vi "GUI PS Main Window.vi"() -> ()   [LabVIEW 2011]
uses:
  Types Definitions/Typer GUI PS.ctl
  <vilib>/Platform/TimedLoop/XDataNode/timing_clust.ctl
  <vilib>/Platform/TimedLoop/XDataNode/nitl_modes.ctl
  <vilib>/Platform/TimedLoop/XDataNode/wakeup.ctl
  Types Definitions/Type Configuration Data (GUI to Controller).ctl
  Types Definitions/Type FOFB Parameters.ctl
  Types Definitions/Type Network Configuration.ctl
  Types Definitions/Type FA Configuration.ctl
  Types Definitions/Type Response Matrix Measurement Configuration.ctl
  Types Definitions/Type Correction Algorithm Configuration.ctl
  Types Definitions/Type Acquisition Network Configuration.ctl
  Types Definitions/Type Actuation Network Configuration.ctl
  Types Definitions/Type Configuration Change Acknowledge (Controller to GUI).ctl
  <vilib>/Platform/TimedLoop/XDataNode/XDataNode.xnode
  <vilib>/Platform/TimedLoop/XDataNode/XDNodeRunTimeDep.lvlib
  Type Definitions.lvlib
  LNLS Control VIs.lvlib
  Misc VIs.lvlib
panel:
  in  "Step de corrente (A)":dbl
  in  "Stop Test":bool
  out "Status":bool
  out "error out":errorcluster
  in  "Step Amplitude OK":bool
  in  "Initialize Test":bool
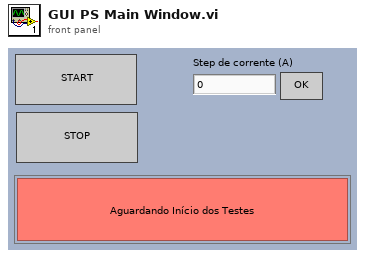
[diagram p1: front panel]
types:
  T1 = enum16{"Idle", "Wait Connection", "Read Data", "Process Data", "Write Data", "Close Connection"}
  T2 = enum16{"Wait Connection", "Read Data", "Write Data", "Close Connection", "Idle"}
  T3 = typedef "Type Definitions.lvlib/Typer GUI PS.ctl" = cluster{"Change Step Value":refnum<notifier>, "Stop VI":refnum<notifier>, "Intialize/Stop Test":refnum<notifier>}
  T4 = typedef "XDNodeRunTimeDep.lvlib/timing_clust.ctl" = cluster{"Expected End [f-1]":u64, "Actual End [f-1]":u64, "Finished Late? [f-1]":bool, "Expected End [i-1]":u64, "Actual End [i-1]":u64, "Finished Late? [i-1]":bool, "Expected Start [i]":u64, "Actual Start [i]":u64, "Expected Start [f]":u64, "Actual Start [f]":u64, "Source Name":string, "Structure Name":string, "Period":i64, "Deadline":i64, "Offset":i64, "Start":i64, "Priority":i32, "Timeout":i32, "Mode":T5, "Wakeup Reason":T6, "Error":errorcluster, "Source Type":string, "Secondary Source Type":string, "Global End Time":u64, "Global Start Time":u64, "Frame Duration":u64, "Iteration Duration":u64, "Assigned CPU":i32, "I/O Scan Engine Mode":u32}
  T5 = typedef "XDNodeRunTimeDep.lvlib/nitl_modes.ctl" = enum32{"No Change", "Process missed periods, maintain original phase", "Discard missed periods, maintain original phase", "Process missed periods, ignore original phase", "Discard missed periods, ignore original phase"}
  T6 = typedef "XDNodeRunTimeDep.lvlib/wakeup.ctl" = enum32{"Normal", "Aborted", "Asynchronous wakeup", "Timing source error", "Timed loop error", "Timeout"}
  T7 = enum16{"Idle Mode", "Error Mode", "Manual Mode", "FOFB Mode", "RMM Mode"}
  T8 = cluster{"Operation Mode":enum16{"Idle Mode", "Error Mode", "Manual Mode", "FOFB Mode", "RMM Mode"}, "Correction Period (usec)":i32, "Beam Energy (MeV)":sgl, "Beam Current (mA)":sgl}
  T9 = typedef "Type Definitions.lvlib/Type Configuration Data (GUI to Controller).ctl" = cluster{"Update Controller Soft Configuration":bool[], "Trigger RT Execution Trace":string[], "Reference Orbit":dbl[], "Request Response Matrix Folder List":bool[], "Request FOFB Parameters":bool[], "FOFB Parameters":T10[]}
  T10 = typedef "Type Definitions.lvlib/Type FOFB Parameters.ctl" = cluster{"Network":T11, "Fast Acquisition":T12, "Response Matrix Measurement":T13, "Correction Algorithm":T14, "Acquisition Network":T15, "Actuation Network":T16}
  T11 = typedef "Type Definitions.lvlib/Type Network Configuration.ctl" = cluster{"FOFB Controller IP":string, "LNLS Control Network IP":string, "LNLS Control Network Power Supplies TCP Port":u16, "LNLS Control Network FOFB Configuration TCP Port":u16, "Data Server TCP Port":u16, "Monitoring Data TCP Port":u16, "Configuration GUI TCP Port":u16, "TCP Listening Timeout":i32}
  T12 = typedef "Type Definitions.lvlib/Type FA Configuration.ctl" = cluster{"Acquisition Period":u32, "Data Buffer Size":u32, "Monitoring Period":u32}
  T13 = typedef "Type Definitions.lvlib/Type Response Matrix Measurement Configuration.ctl" = cluster{"Step Amplitude":dbl, "Time Between Steps":u32, "Step Duration":u32, "Number of Averages":u32}
  T14 = typedef "Type Definitions.lvlib/Type Correction Algorithm Configuration.ctl" = cluster{"Correction Period":u32, "Reference Orbit Path":path, "Response Matrix Path":path, "Correction Matrix Path":path, "Horizontal Correction Factor":dbl, "Vertical Correction Factor":dbl, "Beam Current FOFB Threshold":dbl, "Decouple H-V":bool, "Use Additional BPM LPF":bool, "BPM LPF Cutoff":dbl}
  T15 = typedef "Type Definitions.lvlib/Type Acquisition Network Configuration.ctl" = cluster{"Chassis Name":string, "Variables":cluster{"Variable Name":string, "Matrix Order":u32, "Location":dbl, "Plane":enum8{"H", "V"}, "On Correction":bool}[]}[]
  T16 = typedef "Type Definitions.lvlib/Type Actuation Network Configuration.ctl" = cluster{"Chassis Name":string, "Variables":cluster{"Variable Name":string, "Matrix Order":u32, "RMM Step Factor":dbl, "Plane":enum8{"H", "V"}, "On Correction":bool, "Kc":dbl, "Ti":dbl, "Td":dbl}[]}[]
  T17 = typedef "Type Definitions.lvlib/Type Configuration Change Acknowledge (Controller to GUI).ctl" = cluster{"Request Response Matrix List Folder":string[], "FOFB Parameters":T10[]}
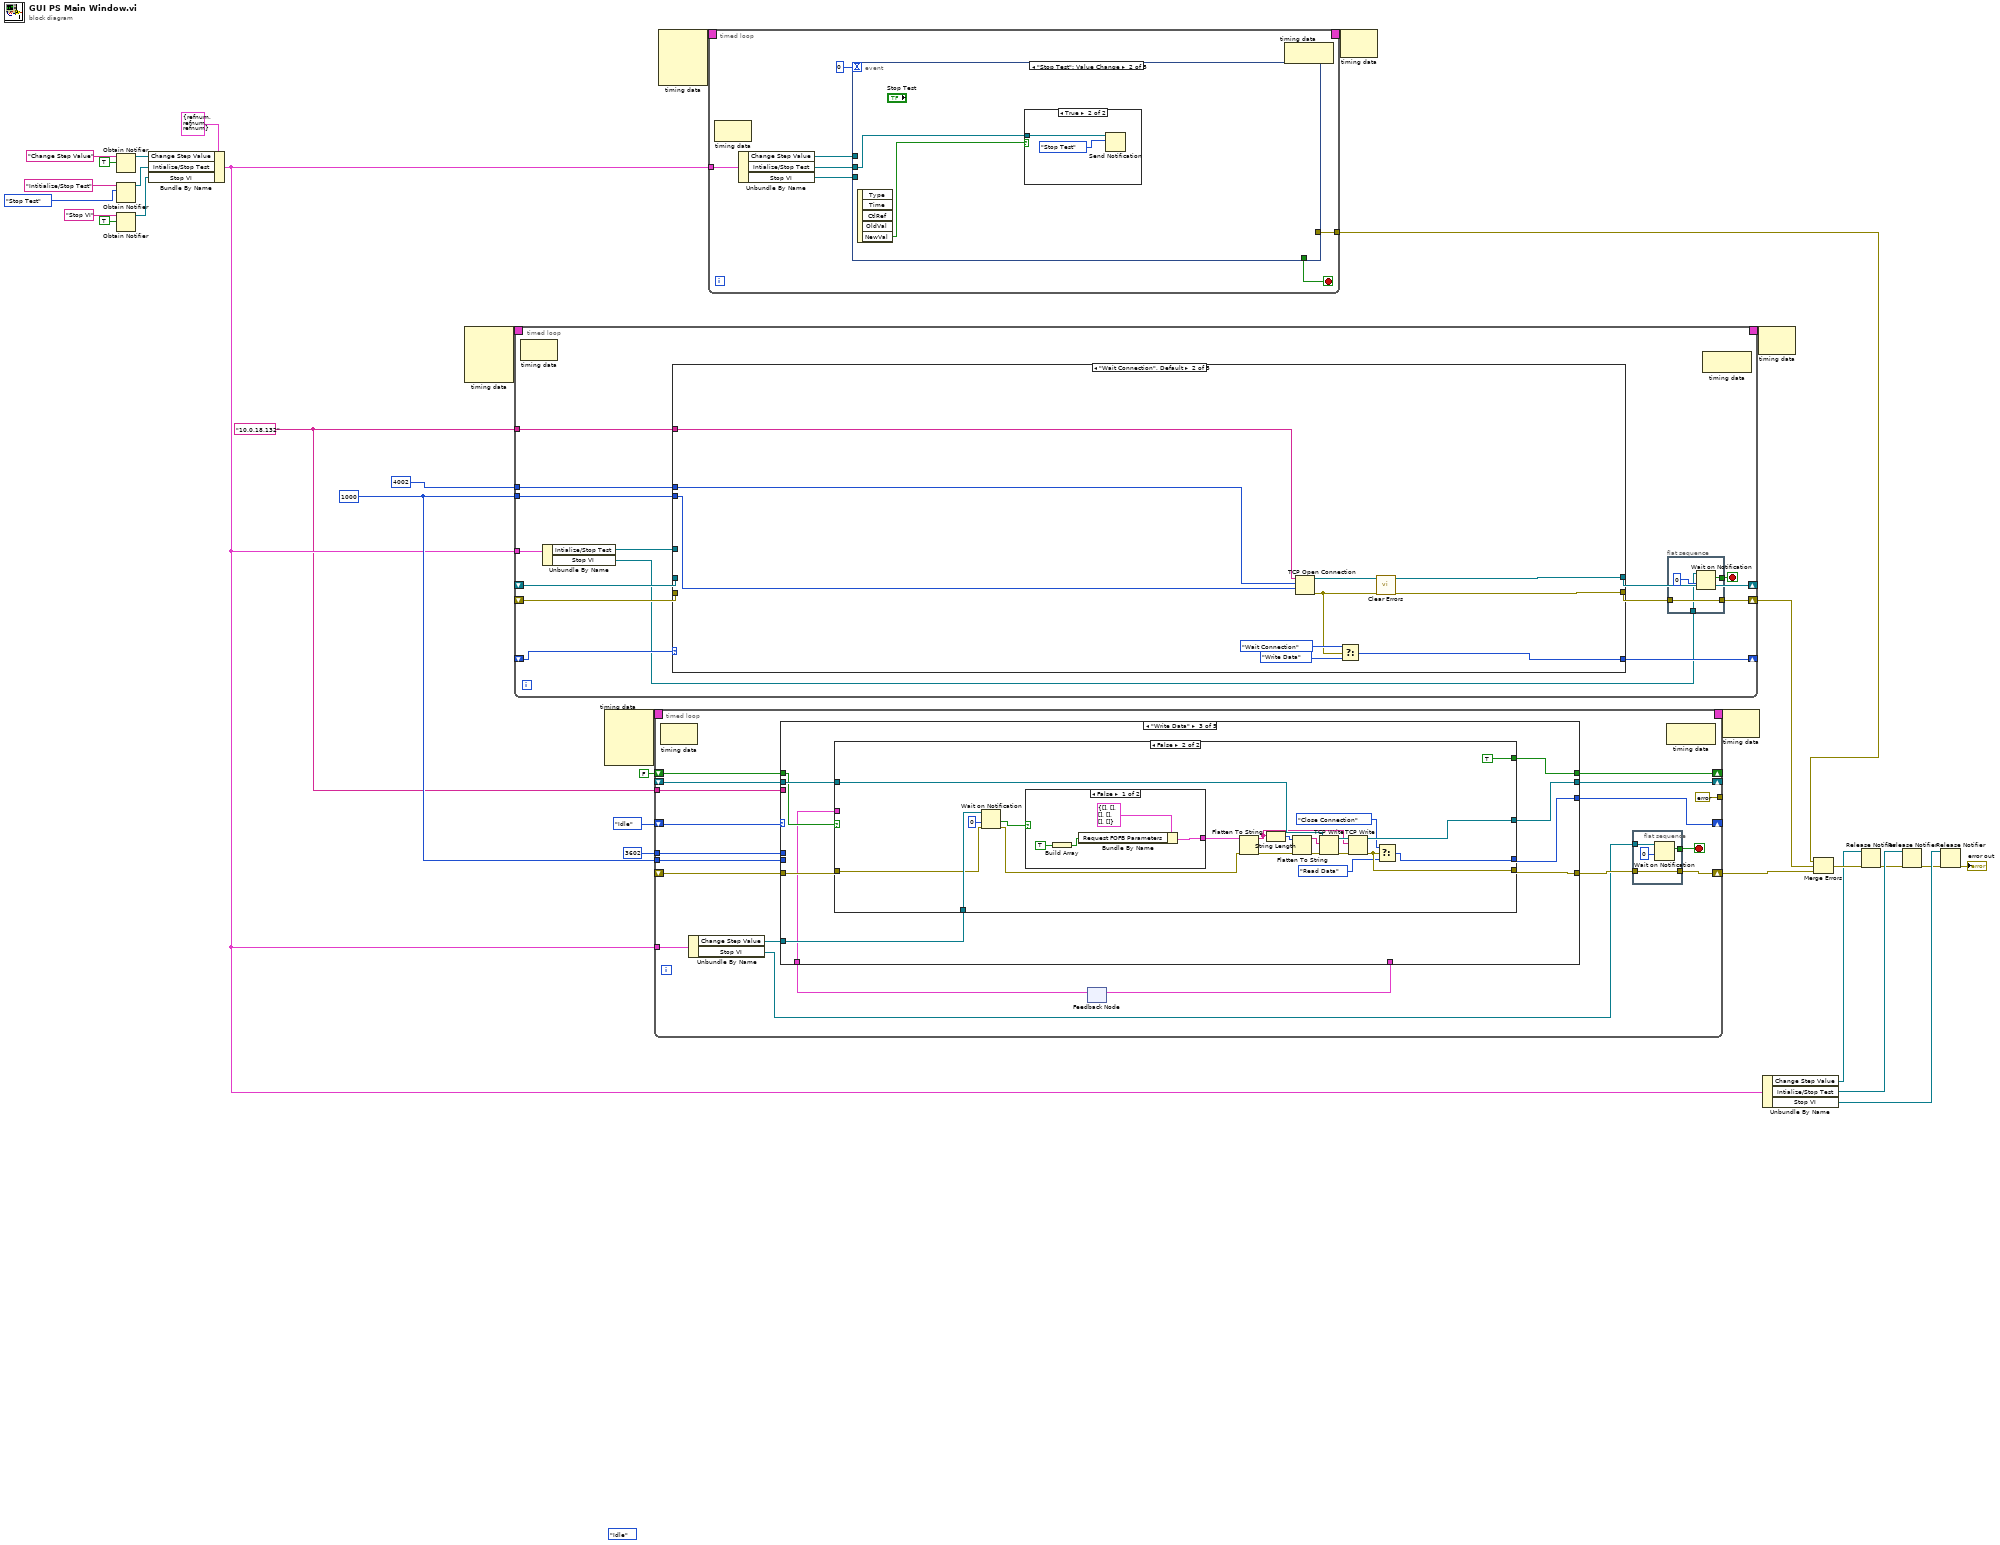
[diagram p0: block diagram]
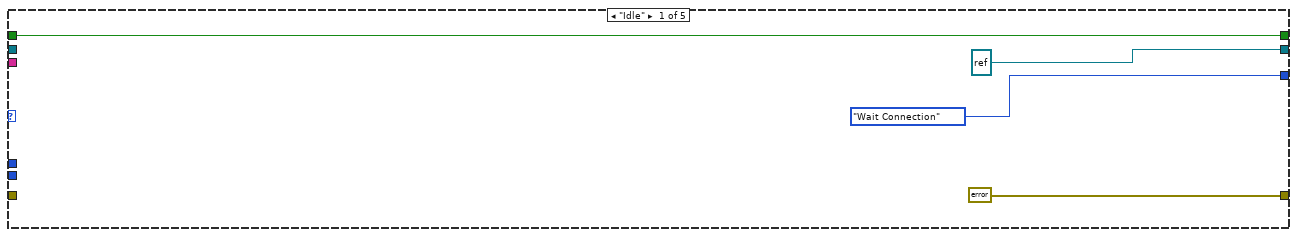
[diagram p2: hidden frame]
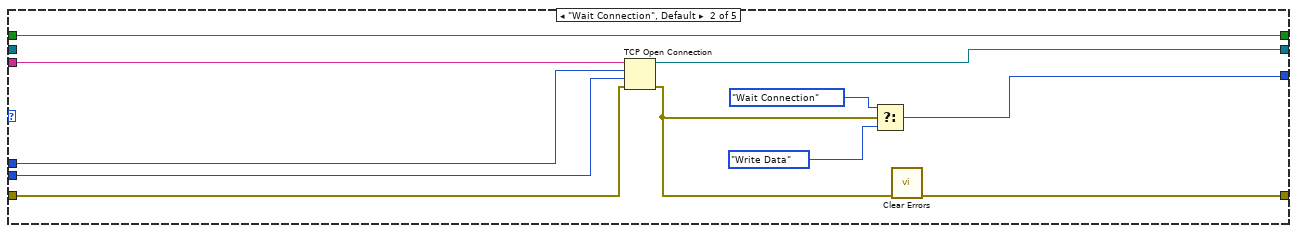
[diagram p3: hidden frame]
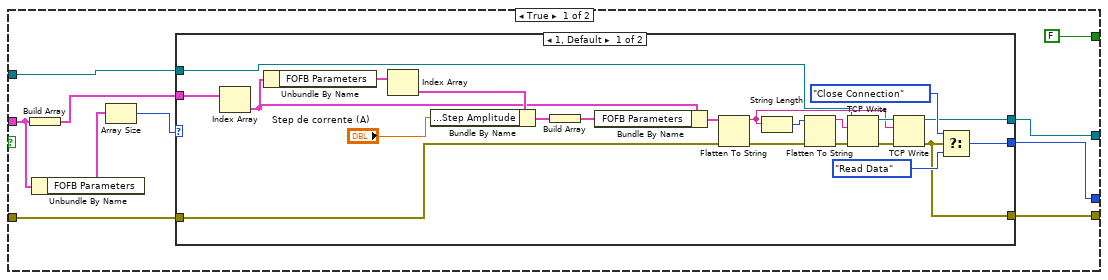
[diagram p4: hidden frame]
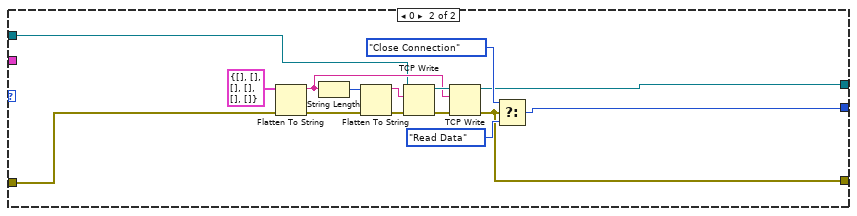
[diagram p5: hidden frame]
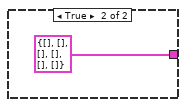
[diagram p6: hidden frame]
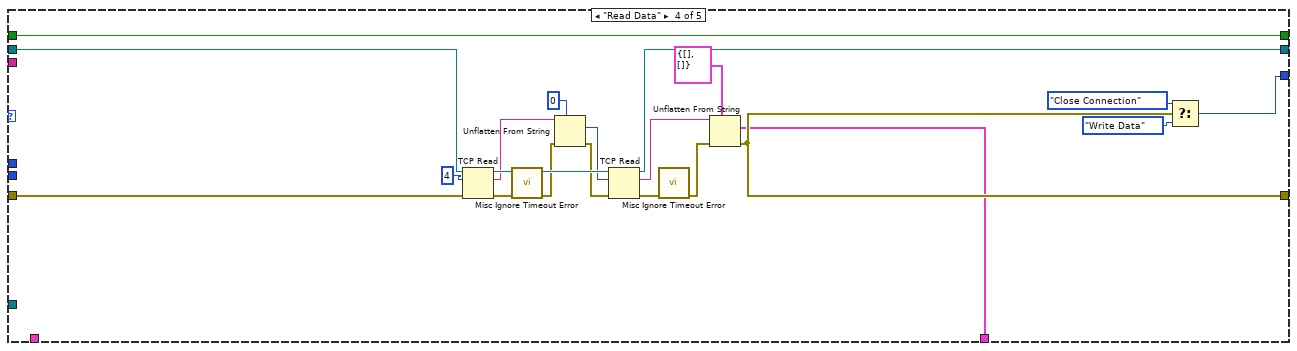
[diagram p7: hidden frame]
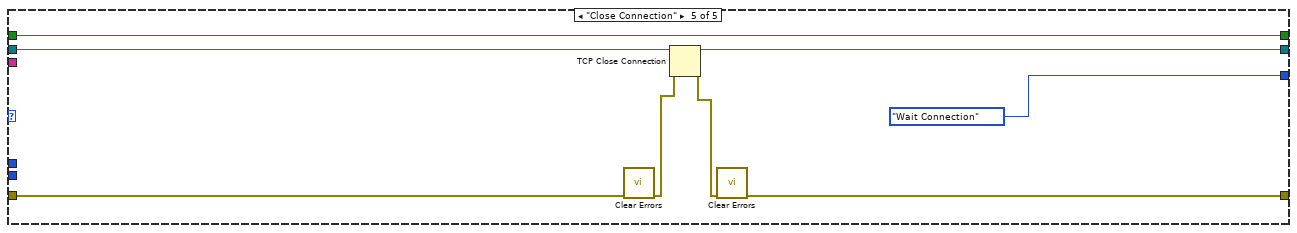
[diagram p8: hidden frame]
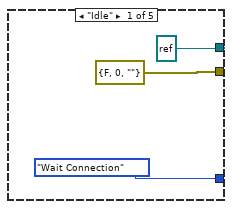
[diagram p9: hidden frame]
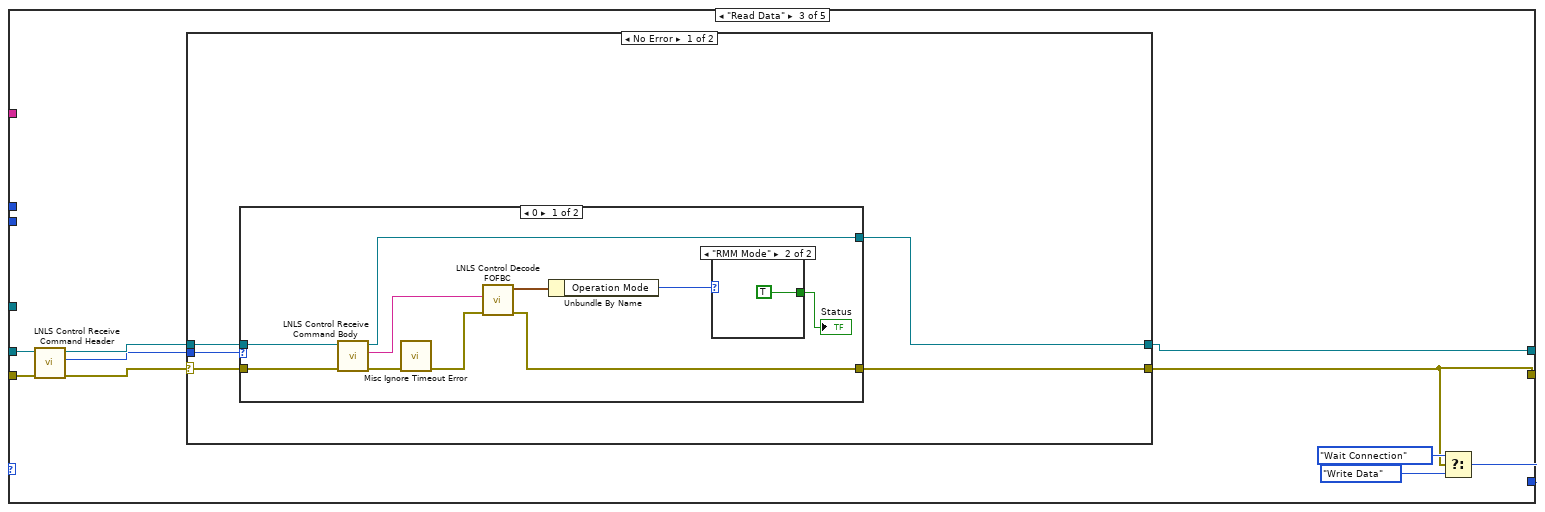
[diagram p10: hidden frame]
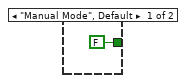
[diagram p11: hidden frame]
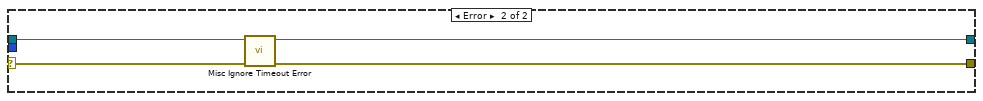
[diagram p13: hidden frame]
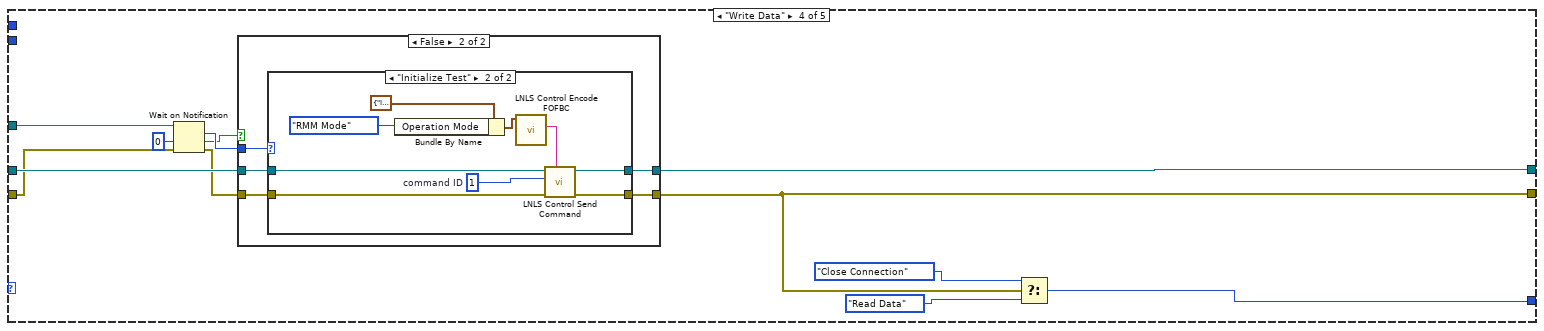
[diagram p14: hidden frame]
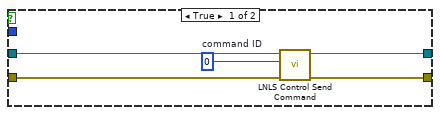
[diagram p15: hidden frame]
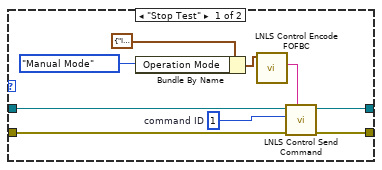
[diagram p16: hidden frame]
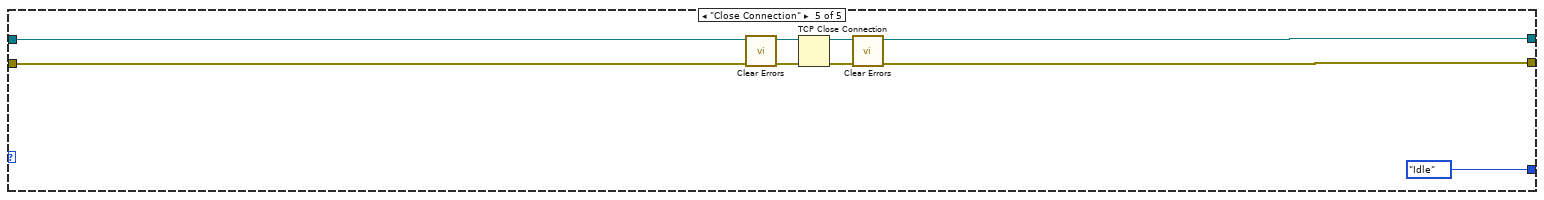
[diagram p17: hidden frame]
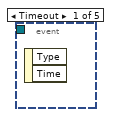
[diagram p18: hidden frame]
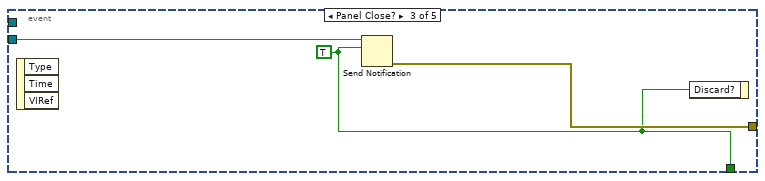
[diagram p20: hidden frame]
diagram:
  (unwired) T2."Idle" ("f")
  w11 = 1000 ("timeout ms (60000)")
  w6 = "10.0.18.132" ("address")
  n1 = Obtain Notifier(name (unnamed)="Change Step Value", notification data type=TRUE) -> (notifier out=w22:refnum<notifier>)  [unwired: 2 in, 2 out]
  n2 = Obtain Notifier(name (unnamed)="Intitialize/Stop Test", notification data type=enum16{"Initialize Test", "Stop Test"}."Stop Test") -> (notifier out=w8:refnum<notifier>)  [unwired: 2 in, 2 out]
  n3 = Obtain Notifier(name (unnamed)="Stop VI", notification data type=TRUE) -> (notifier out=w21:refnum<notifier>)  [unwired: 2 in, 2 out]
  n4 = Bundle By Name(cluster=T3 {"Change Step Value"=refnum, "Stop VI"=refnum, "Intialize/Stop Test"=refnum}, "Change Step Value"=w22, "Intialize/Stop Test"=w8, "Stop VI"=w21) -> (w10:T3)
  n5 = node-c288() -> (w14:T4)  [unwired: 4 in]
  n6 = timed-loop {
    shift-right: [w45] -> _
    shift-left: _ -> [w47]
    shift-right: [w46] -> _
    shift-left: _ -> [w44]
    shift-right: [w38] -> w7
    shift-left: _ -> [w43]
    tunnel: u16 4002 ("remote port or service name") -> [w42]
    tunnel: w11 -> [w40]
    timing: w14 -> [_]
    timing-out: [_] -> w13
    tunnel: w6 -> [w37]
    tunnel: w10 -> [w36]
    stop <- w41 stop-if-true
    n7 = node-c288() -> ()  [unwired: 1 in, 1 out]
    n8 = Unbundle By Name(w36) -> ("Intialize/Stop Test"=w34:refnum<notifier>, "Stop VI"=w35:refnum<notifier>)
    n9 = case shown="\"Wait Connection\", Default" w47 {
      tunnel: [refnum<k5> refnum ("connection ID") w58 w71 w101 w139] -> w46
      tunnel: [errorcluster {"status"=FALSE, "code"=0, "source"=""} ("error out") w56 w63 w103 w136] -> w39
      tunnel: [T2."Wait Connection" w61 w70 w104 T2."Idle"] -> w45
      tunnel: w44 -> [_ _ w68 w102 w140]
      tunnel: w43 -> [_ _ w69 w97 w134]
      tunnel: w42 -> [_ w55 _ _ _]
      tunnel: w40 -> [_ w54 _ _ _]
      tunnel: w37 -> [_ w53 _ _ _]
      tunnel: w34 -> [_ _ _ w100 _]
      frame "Idle" {
      }
      frame "Wait Connection", Default {
        n10 = TCP Open Connection(address=w53, remote port or service name=w55, timeout ms (60000)=w54) -> (connection ID=w58:refnum<k5>, error out=w57:errorcluster)  [unwired: 2 in]
        n11 = Select(t=T2."Wait Connection", s=w57, f=T2."Write Data") -> (s? t:f=w61:T2)
        n12 = call <vilib>:"Clear Errors.vi"("error in (no error)"=w57) -> ("error out"=w56:errorcluster)  [unwired: 6 in]
      }
      frame "Read Data" {
        n13 = call "LNLS Control Receive Command Header.vi"("error in (no error)"=w69, "connection ID"=w68) -> ("error out"=w65:errorcluster, "command ID"=w62:u8, "connection ID out"=w67:refnum<k5>)  [unwired: 7 in]
        n14 = case shown="No Error" w65 {
          selector: w65 -> [w75 w92]
          tunnel: [w74 w93] -> w71
          tunnel: [w72 w91] -> w63
          tunnel: w67 -> [w76 w93]
          tunnel: w62 -> [w73 _]
          frame No Error {
            n15 = case shown="0" w73 {
              tunnel: w76 -> [w86 w90]
              tunnel: w75 -> [w85 w89]
              tunnel: [w84 w90] -> w74
              tunnel: [w83 w89] -> w72
              frame 0 {
                n16 = call "LNLS Control Receive Command Body.vi"("error in (no error)"=w85, "connection ID"=w86) -> ("error out"=w82:errorcluster, "command body"=w80:string, "connection ID out"=w84:refnum<k5>)  [unwired: 6 in, 1 out]
                n17 = call "Misc Ignore Timeout Error.vi"("error in (no error)"=w82) -> ("error out"=w81:errorcluster)  [unwired: 10 in]
                n18 = call "LNLS Control Decode FOFBC.vi"("error in (no error)"=w81, "command body"=w80) -> ("error out"=w83:errorcluster, "LNLS Control FOFB Configuration"=w79:T8)  [unwired: 8 in]
                n19 = Unbundle By Name(w79) -> ("Operation Mode"=w78:T7)
                n20 = case shown="\"RMM Mode\"" w78 {
                  tunnel: [FALSE TRUE] -> w77
                  frame "Manual Mode", Default {
                  }
                  frame "RMM Mode" {
                  }
                }
                "Status" <- w77
              }
              frame 1, Default {
              }
            }
          }
          frame Error {
            n21 = call "Misc Ignore Timeout Error.vi"("error in (no error)"=w92) -> ("error out"=w91:errorcluster)  [unwired: 10 in]
          }
        }
        n22 = Select(t=T2."Wait Connection", s=w63, f=T2."Write Data") -> (s? t:f=w70:T2)
      }
      frame "Write Data" {
        n23 = Wait on Notification(notifier=w100, timeout in ms (-1)=0, error in (no error)=w97) -> (notification=w99:enum16{"Initialize Test", "Stop Test"}, timed out?=w94:bool, error out=w96:errorcluster)  [unwired: 1 in, 1 out]
        n24 = case shown="False" w94 {
          tunnel: [w108 w115] -> w103
          tunnel: w102 -> [w107 w114]
          tunnel: [w106 w113] -> w101
          tunnel: w99 -> [_ w112]
          tunnel: w96 -> [w109 w111]
          frame True {
            w110 = u8 0  # command ID
            n25 = call "LNLS Control Send Command.vi"("error in (no error)"=w109, "command ID"=w110, "connection ID"=w107) -> ("error out"=w108:errorcluster, "connection ID out"=w106:refnum<k5>)  [unwired: 7 in]
          }
          frame False {
            n26 = case shown="\"Initialize Test\"" w112 {
              tunnel: w111 -> [w124 w133]
              tunnel: [w123 w132] -> w115
              tunnel: w114 -> [w122 w131]
              tunnel: [w121 w130] -> w113
              frame "Stop Test" {
                w120 = u8 1  # command ID
                n27 = Bundle By Name(cluster=T8 {"Operation Mode"=enum."Idle Mode", "Correction Period (usec)"=0, "Beam Energy (MeV)"=0.0, "Beam Current (mA)"=0.0} ("LNLS Control FOFB Configuration"), "Operation Mode"=T7."Manual Mode") -> (w116:T8)
                n28 = call "LNLS Control Encode FOFBC.vi"("LNLS Control FOFB Configuration"=w116) -> ("command body"=w119:string)  [unwired: 9 in, 1 out]
                n29 = call "LNLS Control Send Command.vi"("command body"=w119, "error in (no error)"=w124, "command ID"=w120, "connection ID"=w122) -> ("error out"=w123:errorcluster, "connection ID out"=w121:refnum<k5>)  [unwired: 6 in]
              }
              frame "Initialize Test" {
                w129 = u8 1  # command ID
                n30 = Bundle By Name(cluster=T8 {"Operation Mode"=enum."Idle Mode", "Correction Period (usec)"=0, "Beam Energy (MeV)"=0.0, "Beam Current (mA)"=0.0} ("LNLS Control FOFB Configuration"), "Operation Mode"=T7."RMM Mode") -> (w125:T8)
                n31 = call "LNLS Control Encode FOFBC.vi"("LNLS Control FOFB Configuration"=w125) -> ("command body"=w128:string)  [unwired: 9 in, 1 out]
                n32 = call "LNLS Control Send Command.vi"("command body"=w128, "error in (no error)"=w133, "command ID"=w129, "connection ID"=w131) -> ("error out"=w132:errorcluster, "connection ID out"=w130:refnum<k5>)  [unwired: 6 in]
              }
            }
          }
        }
        n33 = Select(t=T2."Close Connection", s=w103, f=T2."Read Data") -> (s? t:f=w104:T2)
      }
      frame "Close Connection" {
        n34 = call <vilib>:"Clear Errors.vi"("error in (no error)"=w134) -> ("error out"=w135:errorcluster)  [unwired: 6 in]
        n35 = TCP Close Connection(connection ID=w140, error in (no error)=w135) -> (connection ID out=w139:refnum<k5>, error out=w137:errorcluster)  [unwired: 1 in]
        n36 = call <vilib>:"Clear Errors.vi"("error in (no error)"=w137) -> ("error out"=w136:errorcluster)  [unwired: 6 in]
      }
    }
    n37 = flat-sequence {
      tunnel: [w143] -> w41
      tunnel: w39 -> [w142]
      tunnel: [w142] -> w38
      tunnel: w35 -> [w141]
      frame #0 {
        n38 = Wait on Notification(notifier=w141, timeout in ms (-1)=0) -> (notification=w143:bool)  [unwired: 2 in, 3 out]
      }
    }
    n39 = node-c288() -> ()  [unwired: 1 in, 1 out]
  }
  n40 = node-c288() -> (w5:T4)  [unwired: 4 in]
  n41 = timed-loop {
    shift-right: [w157] -> w26
    shift-left: _ -> [w161]
    shift-right: [w159] -> _
    shift-left: T1."Idle" ("f") -> [w160]
    shift-right: [w162] -> _
    shift-left: _ -> [w163]
    timing: w5 -> [_]
    timing-out: [_] -> w4
    tunnel: [errorcluster {"status"=FALSE, "code"=0, "source"=""} ("error out")] -> _
    tunnel: w11 -> [w154]
    tunnel: u16 3602 ("remote port or service name") -> [w153]
    tunnel: w6 -> [w152]
    tunnel: w10 -> [w151]
    shift-right: [w145] -> _
    shift-left: FALSE -> [w146]
    stop <- w156 stop-if-true
    n42 = node-c288() -> ()  [unwired: 1 in, 1 out]
    n43 = Unbundle By Name(w151) -> ("Change Step Value"=w149:refnum<notifier>, "Stop VI"=w150:refnum<notifier>)
    n44 = feedback #1() -> (w147:T17)  [unwired: 1 in]
    n45 = case shown="\"Write Data\"" w160 {
      tunnel: [refnum<k5> refnum ("connection ID") w184 w193 w269 w294] -> w162
      tunnel: [T1."Wait Connection" ("f") w183 w188 w271 T1."Wait Connection" ("f")] -> w159
      tunnel: [errorcluster {"status"=FALSE, "code"=0, "source"=""} ("error out") w181 w192 w270 w293] -> w158
      tunnel: w161 -> [_ w180 w189 w272 w288]
      tunnel: w163 -> [_ _ w191 w273 w289]
      tunnel: w154 -> [_ w177 _ _ _]
      tunnel: w153 -> [_ w176 _ _ _]
      tunnel: w152 -> [_ w175 _ _ _]
      tunnel: w149 -> [_ _ w190 _ _]
      tunnel: [_ _ _ w268 _] -> w148
      tunnel: w147 -> [_ _ w185 _ _]
      tunnel: w146 -> [w170 w174 w187 w266 w287]
      tunnel: [w170 w174 w186 w266 w287] -> w145
      frame "Idle" {
      }
      frame "Wait Connection", Default {
        n46 = TCP Open Connection(address=w175, remote port or service name=w176, timeout ms (60000)=w177, error in (no error)=w180) -> (connection ID=w184:refnum<k5>, error out=w182:errorcluster)  [unwired: 1 in]
        n47 = Select(t=T1."Wait Connection" ("f"), s=w182, f=T1."Write Data") -> (s? t:f=w183:T1)
        n48 = call <vilib>:"Clear Errors.vi"("error in (no error)"=w182) -> ("error out"=w181:errorcluster)  [unwired: 6 out]
      }
      frame "Write Data" {
        n49 = case shown="False" w187 {
          tunnel: [w203 w260] -> w193
          tunnel: [w202 w259] -> w192
          tunnel: w191 -> [w200 w258]
          tunnel: w190 -> [_ w256]
          tunnel: w189 -> [w199 w255]
          tunnel: [w201 w243] -> w188
          tunnel: [FALSE TRUE] -> w186
          tunnel: w185 -> [w195 _]
          frame True {
            n50 = Build Array(w195) -> (w196:T17[])
            n51 = Unbundle By Name(w195) -> ("FOFB Parameters"=w194:T10[])
            n52 = Array Size(array=w194) -> (size(s)=w197:i32)
            n53 = case shown="1, Default" w197 {
              tunnel: [w210 w231] -> w203
              tunnel: [w209 w230] -> w202
              tunnel: [w208 w229] -> w201
              tunnel: w200 -> [w207 w228]
              tunnel: w199 -> [w206 w227]
              tunnel: w196 -> [w205 _]
              frame 1, Default {
                n54 = Index Array(array=w205) -> (element=w204:T17)  [unwired: 1 in]
                n55 = Unbundle By Name(w204) -> ("FOFB Parameters"=w216:T10[])
                n56 = Index Array(array=w216) -> (element=w215:T10)  [unwired: 1 in]
                n57 = Bundle By Name(cluster=w215, "Response Matrix Measurement.Step Amplitude"="Step de corrente (A)") -> (w213:T10)
                n58 = Build Array(w213) -> (w212:T10[])
                n59 = Bundle By Name(cluster=w204, "FOFB Parameters"=w212) -> (w211:T17)
                n60 = Flatten To String(anything=w211, error in (no error)=w206) -> (data string=w219:string, error out=w218:errorcluster)  [unwired: 2 in, 1 out]
                n61 = String Length(string=w219) -> (length=w221:i32)
                n62 = Flatten To String(anything=w221, error in (no error)=w218) -> (data string=w220:string, error out=w217:errorcluster)  [unwired: 2 in, 1 out]
                n63 = TCP Write(connection ID=w207, data in=w220, error in (no error)=w217) -> (connection ID out=w223:refnum<k5>, error out=w222:errorcluster)  [unwired: 2 out]
                n64 = TCP Write(connection ID=w223, data in=w219, error in (no error)=w222) -> (connection ID out=w210:refnum<k5>, error out=w209:errorcluster)  [unwired: 2 out]
                n65 = Select(t=T1."Close Connection" ("f"), s=w209, f=T1."Read Data") -> (s? t:f=w208:T1)
              }
              frame 0 {
                n66 = Flatten To String(anything=T9 {"Update Controller Soft Configuration"=[], "Trigger RT Execution Trace"=[], "Reference Orbit"=[], "Request Response Matrix Folder List"=[], "Request FOFB Parameters"=[], "FOFB Parameters"=[]} ("Configuration Data (GUI to Controller)"), error in (no error)=w227) -> (data string=w234:string, error out=w233:errorcluster)  [unwired: 2 in, 1 out]
                n67 = String Length(string=w234) -> (length=w236:i32)
                n68 = Flatten To String(anything=w236, error in (no error)=w233) -> (data string=w235:string, error out=w232:errorcluster)  [unwired: 2 in, 1 out]
                n69 = TCP Write(connection ID=w228, data in=w235, error in (no error)=w232) -> (connection ID out=w238:refnum<k5>, error out=w237:errorcluster)  [unwired: 2 out]
                n70 = TCP Write(connection ID=w238, data in=w234, error in (no error)=w237) -> (connection ID out=w231:refnum<k5>, error out=w230:errorcluster)  [unwired: 2 out]
                n71 = Select(t=T1."Close Connection" ("f"), s=w230, f=T1."Read Data") -> (s? t:f=w229:T1)
              }
            }
          }
          frame False {
            n72 = Wait on Notification(notifier=w256, timeout in ms (-1)=0, error in (no error)=w255) -> (timed out?=w242:bool, error out=w254:errorcluster)  [unwired: 1 in, 2 out]
            n73 = case shown="False" w242 {
              tunnel: [w264 T9 {"Update Controller Soft Configuration"=[], "Trigger RT Execution Trace"=[], "Reference Orbit"=[], "Request Response Matrix Folder List"=[], "Request FOFB Parameters"=[], "FOFB Parameters"=[]} ("Configuration Data (GUI to Controller)")] -> w245
              frame False {
                n74 = Build Array(TRUE) -> (w263:bool[])
                n75 = Bundle By Name(cluster=T9 {"Update Controller Soft Configuration"=[], "Trigger RT Execution Trace"=[], "Reference Orbit"=[], "Request Response Matrix Folder List"=[], "Request FOFB Parameters"=[], "FOFB Parameters"=[]} ("Configuration Data (GUI to Controller)"), "Request FOFB Parameters"=w263) -> (w264:T9)
              }
              frame True {
              }
            }
            n76 = Flatten To String(anything=w245, error in (no error)=w254) -> (data string=w249:string, error out=w247:errorcluster)  [unwired: 2 in, 1 out]
            n77 = String Length(string=w249) -> (length=w251:i32)
            n78 = Flatten To String(anything=w251, error in (no error)=w247) -> (data string=w250:string, error out=w246:errorcluster)  [unwired: 2 in, 1 out]
            n79 = TCP Write(connection ID=w258, data in=w250, error in (no error)=w246) -> (connection ID out=w253:refnum<k5>, error out=w252:errorcluster)  [unwired: 2 out]
            n80 = TCP Write(connection ID=w253, data in=w249, error in (no error)=w252) -> (connection ID out=w260:refnum<k5>, error out=w259:errorcluster)  [unwired: 2 out]
            n81 = Select(t=T1."Close Connection" ("f"), s=w259, f=T1."Read Data") -> (s? t:f=w243:T1)
          }
        }
      }
      frame "Read Data" {
        n82 = TCP Read(connection ID=w273, bytes to read=4, error in (no error)=w272) -> (connection ID out=w286:refnum<k5>, data out=w284:string, error out=w278:errorcluster)  [unwired: 2 in]
        n83 = call "Misc Ignore Timeout Error.vi"("error in (no error)"=w278) -> ("error out"=w276:errorcluster)  [unwired: 10 in]
        n84 = Unflatten From String(type=0 ("bytes to read"), binary string=w284, error in (no error)=w276) -> (value=w282:i32, error out=w275:errorcluster)  [unwired: 2 in, 1 out]
        n85 = TCP Read(connection ID=w286, bytes to read=w282, error in (no error)=w275) -> (connection ID out=w269:refnum<k5>, data out=w281:string, error out=w277:errorcluster)  [unwired: 2 in]
        n86 = call "Misc Ignore Timeout Error.vi"("error in (no error)"=w277) -> ("error out"=w274:errorcluster)  [unwired: 10 in]
        n87 = Unflatten From String(type=T17 {"Request Response Matrix List Folder"=[], "FOFB Parameters"=[]} ("Configuration Change Acknowledge (Controller to GUI)"), binary string=w281, error in (no error)=w274) -> (value=w268:T17, error out=w270:errorcluster)  [unwired: 2 in, 1 out]
        n88 = Select(t=T1."Close Connection" ("f"), s=w270, f=T1."Write Data") -> (s? t:f=w271:T1)
      }
      frame "Close Connection" {
        n89 = call <vilib>:"Clear Errors.vi"("error in (no error)"=w288) -> ("error out"=w292:errorcluster)  [unwired: 6 in]
        n90 = TCP Close Connection(connection ID=w289, error in (no error)=w292) -> (connection ID out=w294:refnum<k5>, error out=w291:errorcluster)  [unwired: 1 in]
        n91 = call <vilib>:"Clear Errors.vi"("error in (no error)"=w291) -> ("error out"=w293:errorcluster)  [unwired: 6 in]
      }
    }
    n92 = feedback-in #1(w148) -> ()
    n93 = flat-sequence {
      tunnel: [w168] -> w156
      tunnel: w158 -> [w167]
      tunnel: [w167] -> w157
      tunnel: w150 -> [w166]
      frame #0 {
        n94 = Wait on Notification(notifier=w166, timeout in ms (-1)=0) -> (notification=w168:bool)  [unwired: 2 in, 3 out]
      }
    }
    n95 = node-c288() -> ()  [unwired: 1 in, 1 out]
  }
  n96 = node-c288() -> (w28:T4)  [unwired: 4 in]
  n97 = timed-loop {
    timing: w28 -> [_]
    timing-out: [_] -> w27
    tunnel: [w299] -> w25
    tunnel: w10 -> [w298]
    stop <- w301 stop-if-true
    n98 = node-c288() -> ()  [unwired: 1 in, 1 out]
    n99 = Unbundle By Name(w298) -> ("Change Step Value"=w297:refnum<notifier>, "Intialize/Stop Test"=w296:refnum<notifier>, "Stop VI"=w295:refnum<notifier>)
    n100 = event shown="[1] \"Stop Test\": Value Change" {
      selector: _ -> [_ _ _ _ _]
      dyn-events: _ -> [_ _ _ _ _]
      timeout: 0 -> [_ _ _ _ _]
      tunnel: [_ _ w306 _ _] -> w301
      tunnel: [_ _ w308 _ _] -> w299
      tunnel: w297 -> [_ _ _ _ w314]
      tunnel: w296 -> [_ w303 _ w310 _]
      tunnel: w295 -> [_ _ w307 _ _]
      event Timeout {
        n101 = event-data() -> ()  [unwired: 1 in, 2 out]
      }
      event "Stop Test": Value Change {
        n102 = event-data() -> ("NewVal"=w302:bool)  [unwired: 1 in, 4 out]
        n103 = case shown="True" w302 {
          tunnel: w303 -> [_ w305]
          frame False {
          }
          frame True {
            n104 = Send Notification(notification=enum16{"Initialize Test", "Stop Test"}."Stop Test", notifier=w305) -> ()  [unwired: 1 in, 2 out]
          }
        }
      }
      event Panel Close? {
        w306 = TRUE
        n105 = event-data() -> ()  [unwired: 1 in, 3 out]
        n106 = Send Notification(notification=w306, notifier=w307) -> (error out=w308:errorcluster)  [unwired: 1 in, 1 out]
        n107 = event-data("Discard?"=w306) -> ()  [unwired: 1 in, 1 out]
      }
      event "Initialize Test": Value Change {
        n108 = event-data() -> ("NewVal"=w309:bool)  [unwired: 1 in, 4 out]
        n109 = case shown="True" w309 {
          tunnel: w310 -> [_ w312]
          frame False {
          }
          frame True {
            n110 = Send Notification(notification=enum16{"Initialize Test", "Stop Test"}."Initialize Test", notifier=w312) -> ()  [unwired: 1 in, 2 out]
          }
        }
      }
      event "Step Amplitude OK": Value Change {
        n111 = event-data() -> ("NewVal"=w313:bool)  [unwired: 1 in, 4 out]
        n112 = case shown="True" w313 {
          selector: w313 -> [_ w315]
          tunnel: w314 -> [_ w316]
          frame False {
          }
          frame True {
            n113 = Send Notification(notification=w315, notifier=w316) -> ()  [unwired: 1 in, 2 out]
          }
        }
      }
    }
    n114 = node-c288() -> ()  [unwired: 1 in, 1 out]
  }
  n115 = node-c288(w27) -> ()  [unwired: 1 out]
  n116 = node-c288(w4) -> ()  [unwired: 1 out]
  n117 = node-c288(w13) -> ()  [unwired: 1 out]
  n118 = Unbundle By Name(w10) -> ("Change Step Value"=w20:refnum<notifier>, "Intialize/Stop Test"=w19:refnum<notifier>, "Stop VI"=w18:refnum<notifier>)
  n119 = Merge Errors(w25, w7, w26) -> (w24:errorcluster)
  n120 = Release Notifier(notifier=w20, error in (no error)=w24) -> (error out=w17:errorcluster)  [unwired: 1 in, 2 out]
  n121 = Release Notifier(notifier=w19, error in (no error)=w17) -> (error out=w16:errorcluster)  [unwired: 1 in, 2 out]
  n122 = Release Notifier(notifier=w18, error in (no error)=w16) -> (error out=→"error out":errorcluster)  [unwired: 1 in, 2 out]
